vi "getstamp.vi"(8 "error in":errorcluster, 10 "Array":string[](array[string]), 11 "Gantry in":refnum<class "Gantry.lvclass">) -> (0 "error out":errorcluster, 3 "Gantry out":refnum<class "Gantry.lvclass">)   [LabVIEW 2017]
uses:
  Shared Components/Gantry Class/Gantry.lvclass
  Shared Components/FlexWorktable/FlexWorktable.lvclass
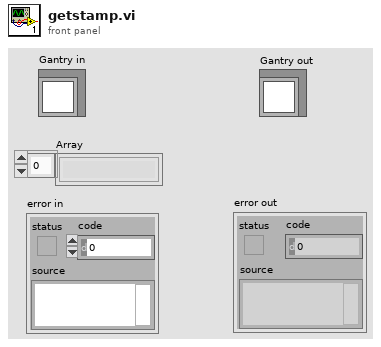
[diagram p1: front panel]
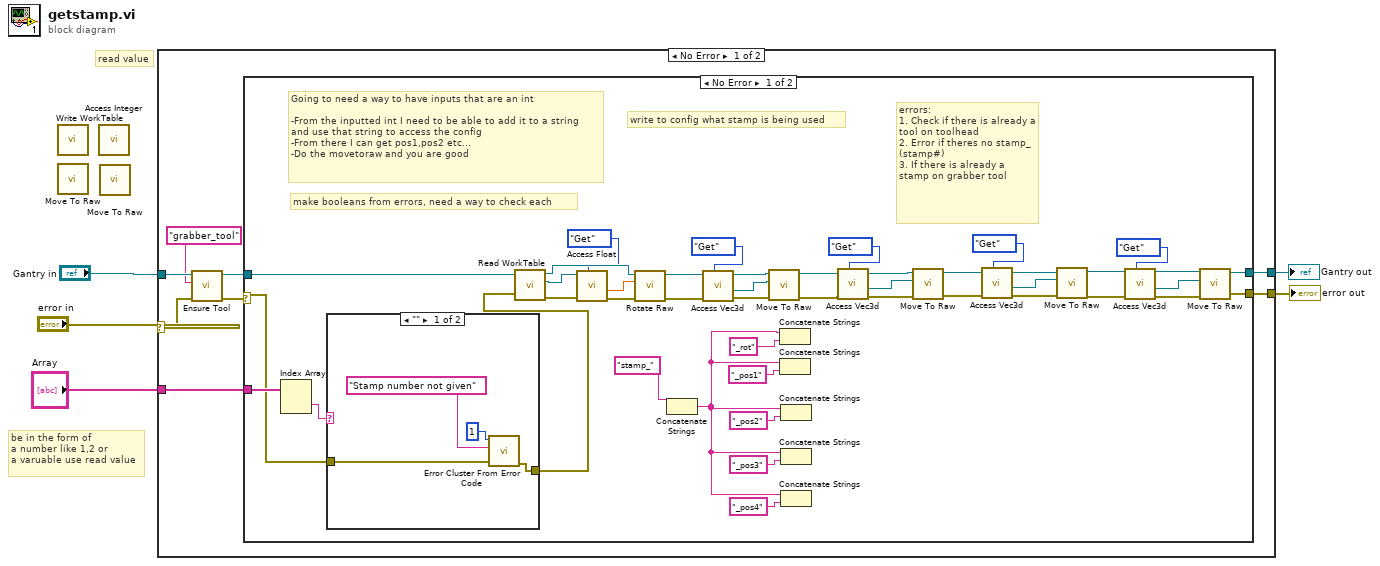
[diagram p0: block diagram]
diagram:
  # "be in the form of\na number like 1,2 or \na varuable use read value"
  # "read value"
  n1 = call-dynamic "Write WorkTable.vi"() -> ()  [unwired: 10 in, 2 out]
  n2 = call-dynamic "Move To Raw.vi"() -> ()  [unwired: 10 in, 2 out]
  n3 = call-dynamic "Access Integer.vi"() -> ()  [unwired: 9 in, 3 out]
  n4 = call-dynamic "Move To Raw.vi"() -> ()  [unwired: 10 in, 2 out]
  n5 = case shown="No Error" "error in" {
    selector: "error in" -> [w12 _]
    tunnel: "Gantry in" -> [w13 _]
    tunnel: "Array" -> [w8 _]
    tunnel: [w7 _] -> w2
    tunnel: [w6 _] -> w1
    frame No Error {
      n6 = call "Ensure Tool.vi"("error in (no error)"=w12, "Tool Name"="grabber_tool", "Gantry in"=w13) -> ("error out"=w10:errorcluster, "Gantry out"=w9:refnum<class "Gantry.lvclass">)  [unwired: 7 in]
      n7 = case shown="No Error" w10 {
        selector: w10 -> [w14 _]
        tunnel: w9 -> [w28 _]
        tunnel: w8 -> [w25 _]
        tunnel: [w27 _] -> w7
        tunnel: [w26 _] -> w6
        frame No Error {
          # "write to config what stamp is being used"
          # "errors:\n1. Check if there is already a tool on toolhead\n2. Error if theres no stamp_(stamp#)\n3. If there is already a stamp on grabber tool"
          # "make booleans from errors, need a way to check each"
          # "Going to need a way to have inputs that are an int\n\n-From the inputted int I need to be able to add it to a string\nand use that string to access the config\n-From there I can get pos1,pos2 etc...\n-Do the movetoraw and you are good"
          n8 = Index Array(array=w25) -> (element #1=w24:string)  [unwired: 2 in, 1 out]
          n9 = case shown="\"\"" w24 {
            tunnel: w14 -> [w56 _]
            tunnel: [w55 _] -> w15
            frame "" {
              n10 = call <vilib>:"Error Cluster From Error Code.vi"("error in (no error)"=w56, "error message (\"\")"="Stamp number not given" ("error message (\"\")"), "error code (0)"=1) -> ("error out"=w55:errorcluster)  [unwired: 6 in]
            }
            frame Default {
            }
          }
          n11 = call-dynamic "Read WorkTable.vi"("error in"=w15, "Gantry Class in"=w28) -> ("error out"=w52:errorcluster, "Worktable"=w53:refnum<class "FlexWorktable.lvclass">, "Gantry Class out"=w54:refnum<class "Gantry.lvclass">)  [unwired: 7 in]
          n12 = call-dynamic "Access Float.vi"("Get/Set"=enum16{"Get", "Set"}."Get", "error in (no error)"=w52, "FlexWorktable in"=w53) -> ("error out"=w34:errorcluster, "Value out"=w51:dbl)  [unwired: 6 in, 1 out]
          n13 = call-dynamic "Rotate Raw.vi"("error in"=w34, "position(deg)"=w51, "Gantry in"=w54) -> ("error out"=w49:errorcluster, "Gantry out"=w50:refnum<class "Gantry.lvclass">)  [unwired: 7 in]
          n14 = Concatenate Strings("stamp_") -> (w18:string, w16:string)
          n15 = call-dynamic "Access Vec3d.vi"("Get/Set"=enum16{"Get", "Set"}."Get", "error in (no error)"=w49) -> ("error out"=w35:errorcluster, "Value out"=w36:refnum<class "Vec3d.lvclass">)  [unwired: 7 in, 1 out]
          n16 = call-dynamic "Move To Raw.vi"("error in"=w35, "Destination"=w36, "Gantry in"=w50) -> ("error out"=w38:errorcluster, "Gantry out"=w40:refnum<class "Gantry.lvclass">)  [unwired: 7 in]
          n17 = Concatenate Strings(w18, "_rot" ("string")) -> ()  [unwired: 1 out]
          n18 = Concatenate Strings(w18, "_pos1" ("string")) -> ()  [unwired: 1 out]
          n19 = Concatenate Strings(w18, "_pos2" ("string")) -> ()  [unwired: 1 out]
          n20 = Concatenate Strings(w18, "_pos3" ("string")) -> ()  [unwired: 1 out]
          n21 = Concatenate Strings(w18, "_pos4" ("string")) -> ()  [unwired: 1 out]
          n22 = call-dynamic "Access Vec3d.vi"("Get/Set"=enum16{"Get", "Set"}."Get", "error in (no error)"=w38) -> ("error out"=w37:errorcluster, "Value out"=w39:refnum<class "Vec3d.lvclass">)  [unwired: 7 in, 1 out]
          n23 = call-dynamic "Move To Raw.vi"("error in"=w37, "Destination"=w39, "Gantry in"=w40) -> ("error out"=w43:errorcluster, "Gantry out"=w44:refnum<class "Gantry.lvclass">)  [unwired: 7 in]
          n24 = call-dynamic "Access Vec3d.vi"("Get/Set"=enum16{"Get", "Set"}."Get", "error in (no error)"=w43) -> ("error out"=w41:errorcluster, "Value out"=w42:refnum<class "Vec3d.lvclass">)  [unwired: 7 in, 1 out]
          n25 = call-dynamic "Move To Raw.vi"("error in"=w41, "Destination"=w42, "Gantry in"=w44) -> ("error out"=w47:errorcluster, "Gantry out"=w48:refnum<class "Gantry.lvclass">)  [unwired: 7 in]
          n26 = call-dynamic "Access Vec3d.vi"("Get/Set"=enum16{"Get", "Set"}."Get", "error in (no error)"=w47) -> ("error out"=w45:errorcluster, "Value out"=w46:refnum<class "Vec3d.lvclass">)  [unwired: 7 in, 1 out]
          n27 = call-dynamic "Move To Raw.vi"("error in"=w45, "Destination"=w46, "Gantry in"=w48) -> ("error out"=w26:errorcluster, "Gantry out"=w27:refnum<class "Gantry.lvclass">)  [unwired: 7 in]
        }
        frame Error {
          # "Tool already loaded"
        }
      }
    }
    frame Error {
    }
  }
  "Gantry out" <- w2
  "error out" <- w1
